vi "LogFileGlobal.vi"(7 "Action":T1, 8 "Error In":errorcluster, 10 "CSV String":string, 11 "Path":path) -> (0 "Error Out":errorcluster, 3 "Size (bytes)":i64)   [LabVIEW 2012]
uses:
  LogFileGlobalAction.ctl
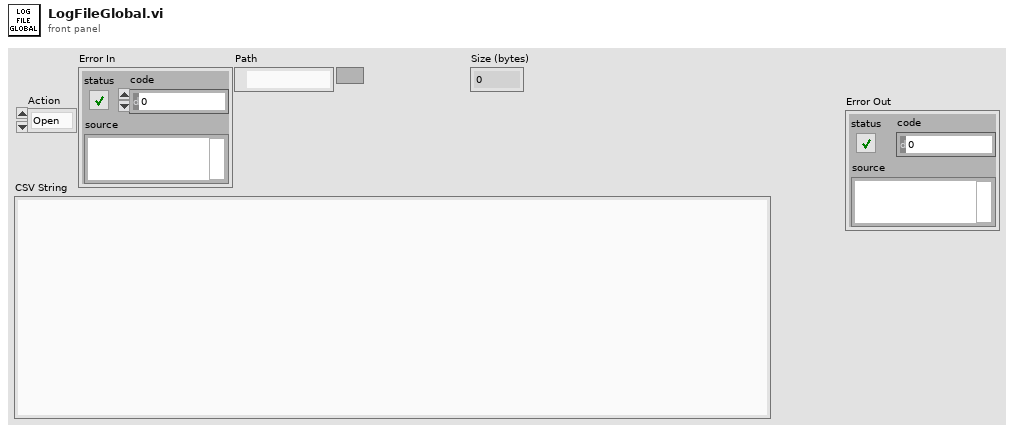
[diagram p1: front panel]
types:
  T1 = typedef "LogFileGlobalAction.ctl" = enum16{"Open", "Write", "Size", "Close"}
  T2 = enum16{"open", "replace", "create", "open or create", "replace or create", "replace or create with confirmation"}
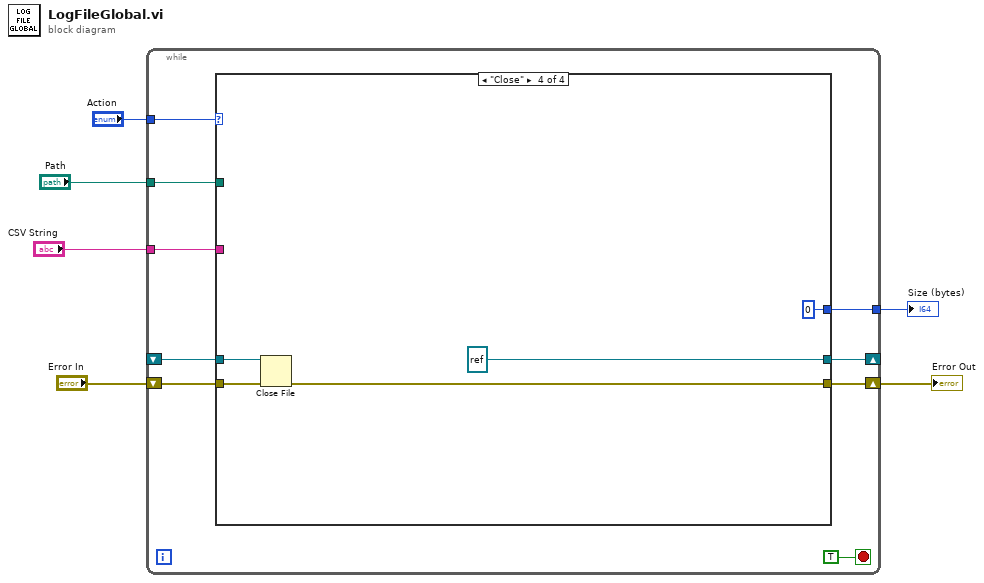
[diagram p0: block diagram]
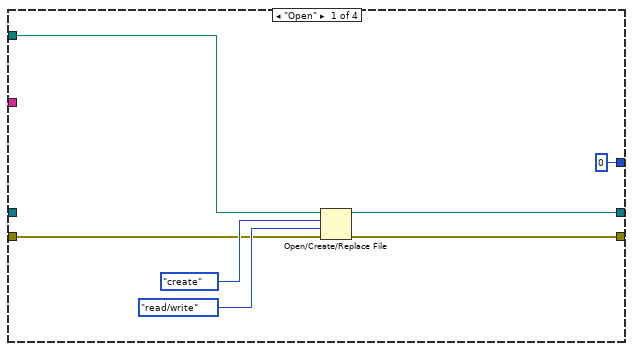
[diagram p2: hidden frame]
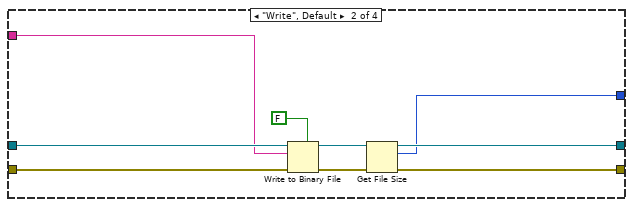
[diagram p3: hidden frame]
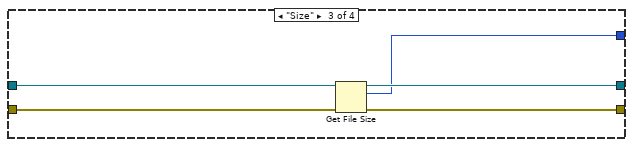
[diagram p4: hidden frame]
diagram:
  n1 = while {
    shift-right: [w14] -> _
    shift-left: _ -> [w13]
    tunnel: "Action" -> [w12]
    shift-right: [w11] -> w5
    shift-left: "Error In" -> [w10]
    tunnel: "CSV String" -> [w9]
    tunnel: "Path" -> [w8]
    tunnel: [w7] -> w1
    stop <- TRUE stop-if-true
    n2 = case shown="\"Close\"" w12 {
      tunnel: [w20 w26 w33 refnum<file> refnum ("refnum out")] -> w14
      tunnel: w13 -> [_ w30 w36 w41]
      tunnel: [w18 w25 w34 w39] -> w11
      tunnel: w10 -> [w19 w29 w35 w38]
      tunnel: w9 -> [_ w28 _ _]
      tunnel: w8 -> [w17 _ _ _]
      tunnel: [i64 0 ("size (in bytes)") w23 w32 i64 0 ("size (in bytes)")] -> w7
      frame "Open" {
        n3 = Open/Create/Replace File(file path (use dialog)=w17, error in=w19, operation (0:open)=T2."create", access (0:read/write)=enum16{"read/write", "read-only", "write-only"}."read/write") -> (refnum out=w20:refnum<file>, error out=w18:errorcluster)  [unwired: 2 in, 1 out]
      }
      frame "Write", Default {
        n4 = Write to Binary File(file (use dialog)=w30, data=w28, error in=w29, 5:FALSE ("prepend array or string size? (T)")) -> (refnum out=w27:refnum<file>, error out=w24:errorcluster)  [unwired: 2 in, 1 out]
        n5 = Get File Size(file=w27, error in=w24) -> (refnum out=w26:refnum<file>, size (in bytes)=w23:i64, 0:w25:errorcluster)
      }
      frame "Size" {
        n6 = Get File Size(file=w36, error in=w35) -> (refnum out=w33:refnum<file>, size (in bytes)=w32:i64, 0:w34:errorcluster)
      }
      frame "Close" {
        n7 = Close File(refnum=w41, error in=w38) -> (error out=w39:errorcluster)  [unwired: 1 out]
      }
    }
  }
  "Error Out" <- w5
  "Size (bytes)" <- w1
